vi "AssertValueByFocusIndex.vi"(0 "VI Reference In":refnum<vi>, 1 "Test Label":string, 2 "delimiter (>>)":string=">>", 3 "Assert Only? (F)":bool, 5 "Control Path":string, 7 "Focus Index":i32, 11 "Error In":errorcluster, 12 "Assert Interval(10 ms)":u32=10, 13 "Timeout(5 sec)":dbl=5.0) -> (4 "VI Reference Out":refnum<vi>, 6 "Asserted Value":i32, 15 "Error Out":errorcluster)   [LabVIEW 2016, in "Drona.lvlib" / "AssertControlValue.lvlib" / "AssertMCListbox.lvlib"]
doc: "Asserts if the focus item index on multi-column listbox control is equal.\n\nThe input control name is given as a string, incase of the path, use delimiters in between the path.\nThis VI gets the control value until the value is equal to the input value."
uses:
  AssertMCListbox.lvlib
  Get/GetControlRef/GetControlRefByPath.vi
  <vilib>/addons/_JKI Toolkits/Caraya/classes/Assert/Assert Equal Value_Variant.vi
  <vilib>/Utility/error.llb/Error Cluster From Error Code.vi
  <vilib>/ErrorRing/Error Ring.xnode
  <vilib>/addons/_JKI Toolkits/Caraya/classes/Assert/Assert.lvclass
  Get/GetControlRef/GetControlRef.lvlib
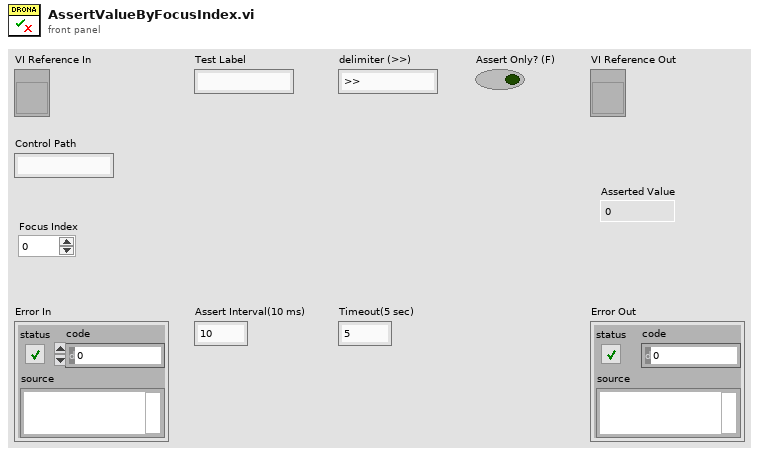
[diagram p1: front panel]
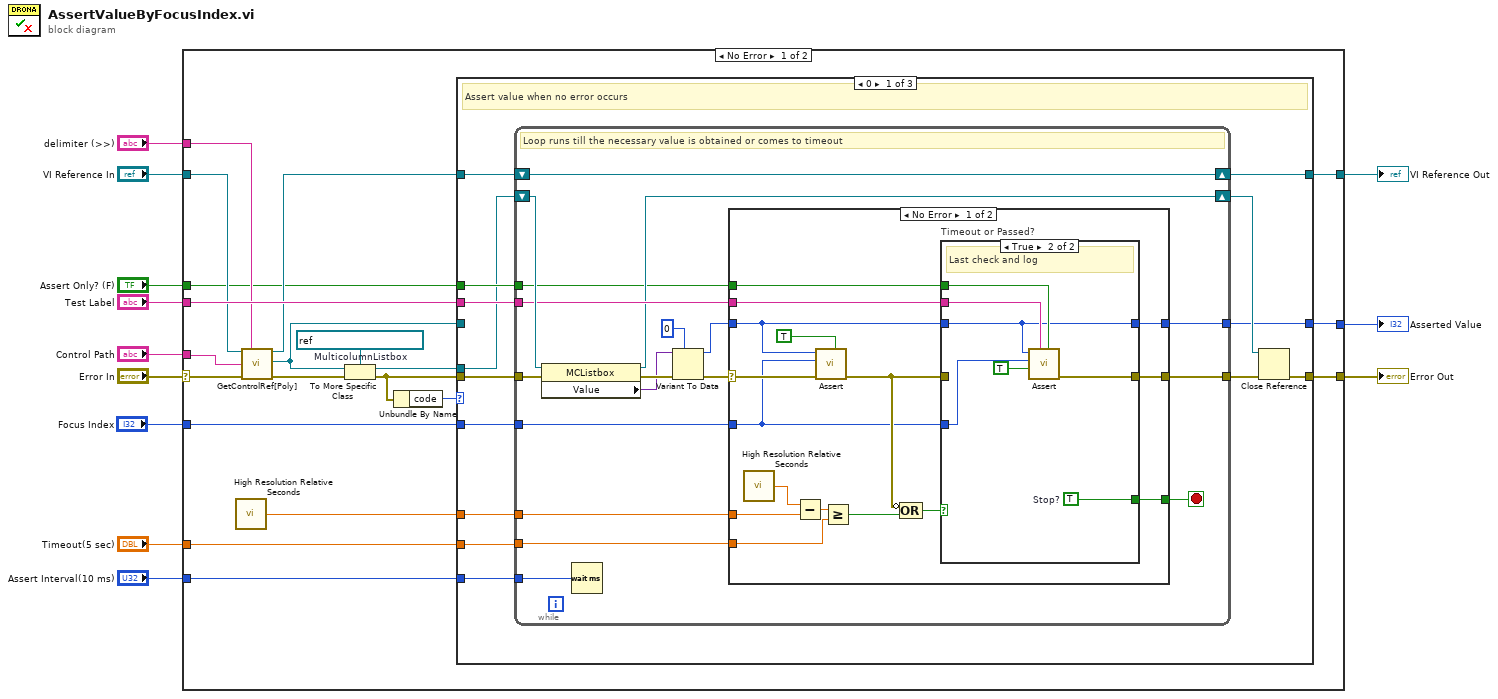
[diagram p0: block diagram]
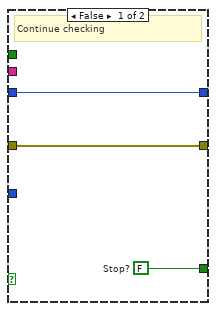
[diagram p2: hidden frame]
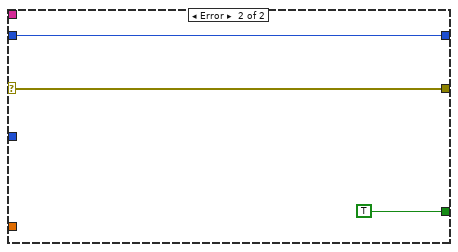
[diagram p3: hidden frame]
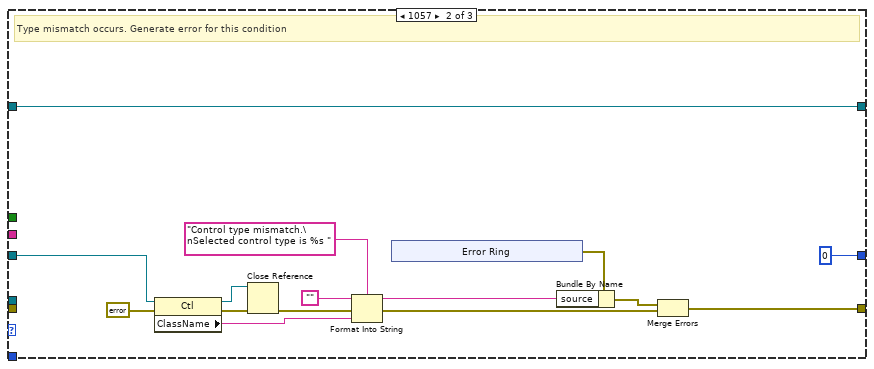
[diagram p4: hidden frame]
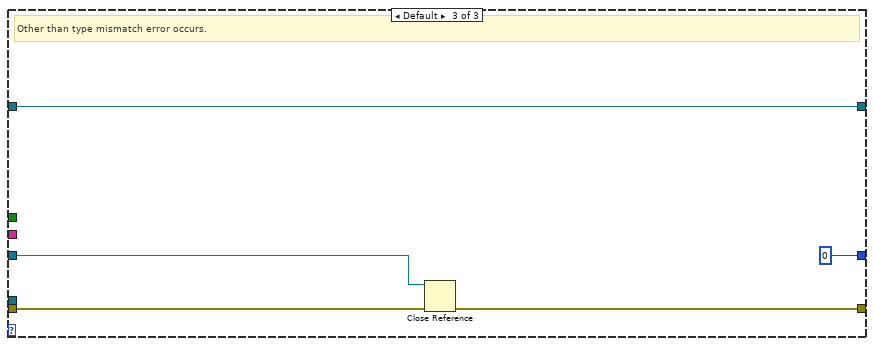
[diagram p5: hidden frame]
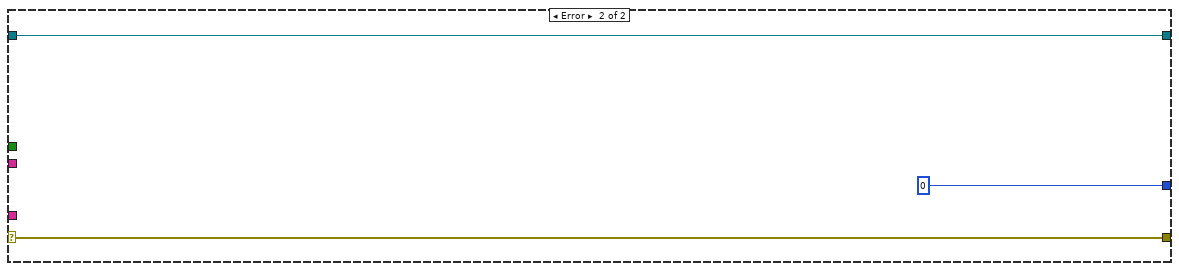
[diagram p6: hidden frame]
diagram:
  n1 = case shown="No Error" "Error In" {
    selector: "Error In" -> [w27 w121]
    tunnel: "Timeout(5 sec)" -> [w32 _]
    tunnel: [w31 w120] -> w11
    tunnel: "Focus Index" -> [w30 _]
    tunnel: [w21 w121] -> w10
    tunnel: "Assert Interval(10 ms)" -> [w29 _]
    tunnel: "Test Label" -> [w28 _]
    tunnel: "VI Reference In" -> [w26 w120]
    tunnel: "Control Path" -> [w25 _]
    tunnel: "delimiter (>>)" -> [w20 _]
    tunnel: "Assert Only? (F)" -> [w19 _]
    tunnel: [w18 0] -> w2
    frame No Error {
      w17 = refnum<vi> refnum  # MulticolumnListbox
      n2 = call <vilib>:"High Resolution Relative Seconds.vi"() -> ("relative seconds"=w24:dbl)
      n3 = call-poly "GetControlRef[Poly].vi"("VI Reference In"=w26, "delimiter (>>)"=w20, "Control Path"=w25, "error In"=w27) -> ("VI Reference Out"=w22:refnum<vi>, "Ctl Refnum"=w13:refnum<vi>, "error out"=w23:errorcluster)  [unwired: 9 in]
      n4 = To More Specific Class(target class=w17, reference=w13, error in=w23) -> (specific class reference=w16:refnum<vi>, error out=w15:errorcluster)
      n5 = Unbundle By Name(w15) -> ("code"=w14:i32)
      n6 = case shown="0" w14 {
        tunnel: w32 -> [w46 _ _]
        tunnel: [w45 w96 w116] -> w31
        tunnel: w30 -> [w44 _ _]
        tunnel: w29 -> [w42 _ _]
        tunnel: w28 -> [w41 _ _]
        tunnel: w24 -> [w40 _ _]
        tunnel: w22 -> [w39 w96 w116]
        tunnel: [w38 w97 w115] -> w21
        tunnel: w19 -> [w36 _ _]
        tunnel: [w35 0 0] -> w18
        tunnel: w15 -> [w34 _ w118]
        tunnel: w16 -> [w33 _ _]
        tunnel: w13 -> [_ w94 w114]
        frame 0 {
          # "Assert value when no error occurs"
          n7 = while {
            tunnel: w44 -> [w51]
            tunnel: w46 -> [w63]
            tunnel: w40 -> [w64]
            tunnel: w34 -> [w58]
            tunnel: [w61] -> w43
            tunnel: w42 -> [w59]
            tunnel: w41 -> [w55]
            shift-right: [w56] -> w45
            shift-left: w39 -> [w56]
            shift-right: [w54] -> w37
            shift-left: w33 -> [w57]
            tunnel: w36 -> [w53]
            tunnel: [w52] -> w35
            stop <- w62 stop-if-true
            # "Loop runs till the necessary value is obtained or comes to timeout"
            n8 = property on="Property Node" class="MCListbox"(reference=w57, error in=w58) -> (reference out=w54:refnum<vi>, error out=w60:errorcluster, "Value"=w49:variant)
            n9 = Wait (ms)(milliseconds to wait=w59) -> ()  [unwired: 1 out]
            n10 = Variant To Data(error in=w60, type=0, Variant=w49) -> (data=w47:i32, error out=w50:errorcluster)
            n11 = case shown="No Error" w50 {
              selector: w50 -> [w76 w93]
              tunnel: w64 -> [w80 _]
              tunnel: w63 -> [w77 _]
              tunnel: [w67 TRUE] -> w62
              tunnel: [w68 w93] -> w61
              tunnel: w51 -> [w69 _]
              tunnel: w47 -> [w70 w91]
              tunnel: w55 -> [w75 _]
              tunnel: w53 -> [w66 _]
              tunnel: [w65 w91] -> w52
              frame No Error {
                n12 = call <vilib>:"High Resolution Relative Seconds.vi"() -> ("relative seconds"=w79:dbl)
                n13 = Subtract(x=w79, y=w80) -> (x-y=w78:dbl)
                n14 = call-poly <vilib>:"Assert.vi"("Assert Only? (F)"=TRUE, "error in (no error)"=w76, "Y"=w69, "X"=w70) -> ("error out"=w73:errorcluster)  [unwired: 7 in]
                n15 = Greater Or Equal?(x=w78, y=w77) -> (x >= y?=w74:bool)
                n16 = Compound Arithmetic op=OR(invert w73, w74) -> (w72:bool)
                n17 = case "Timeout or Passed?" shown="True" w72 {
                  tunnel: w73 -> [w83 _]
                  tunnel: w69 -> [_ w89]
                  tunnel: w70 -> [w81 w84]
                  tunnel: w75 -> [_ w90]
                  tunnel: [w83 w88] -> w68
                  tunnel: [w82 w87] -> w67
                  tunnel: w66 -> [_ w85]
                  tunnel: [w81 w84] -> w65
                  frame False {
                    w82 = FALSE  # Stop?
                    # "Continue checking"
                  }
                  frame True {
                    w87 = TRUE  # Stop?
                    # "Last check and log"
                    n18 = call-poly <vilib>:"Assert.vi"("Assert Only? (F)"=w85, "Label"=w90, "Register with caller test (F)"=TRUE, "Y"=w89, "X"=w84) -> ("error out"=w88:errorcluster)  [unwired: 6 in]
                  }
                }
              }
              frame Error {
              }
            }
          }
          n19 = Close Reference(reference=w37, error in (no error)=w43) -> (error out=w38:errorcluster)
        }
        frame 1057 {
          # "Type mismatch occurs. Generate error for this condition"
          n20 = property class="Ctl"(reference=w94, error in=errorcluster {"status"=FALSE, "code"=0, "source"=""} ("error out")) -> (reference out=w98:refnum<vi>, error out=w108:errorcluster, "ClassName"=w105:string)
          n21 = Close Reference(reference=w98, error in (no error)=w108) -> (error out=w99:errorcluster)
          n22 = Format Into String(format string="Control type mismatch.\nSelected control type is %s ", initial string="", error in=w99, w105) -> (resulting string=w102:string, error out=w100:errorcluster)
          n23 = xnode "Error Ring"() -> ("error out"=w103:errorcluster)
          n24 = Bundle By Name(cluster=w103, "source"=w102) -> (w101:errorcluster)
          n25 = Merge Errors(w101, w100) -> (w97:errorcluster)
        }
        frame Default {
          # "Other than type mismatch error occurs."
          n26 = Close Reference(reference=w114, error in (no error)=w118) -> (error out=w115:errorcluster)
        }
      }
    }
    frame Error {
    }
  }
  "Error Out" <- w10
  "VI Reference Out" <- w11
  "Asserted Value" <- w2
